vi "collisionTest.vi"(0 "Game in":refnum<class "Game.lvclass">, 1 "TestParameters":T7, 2 "replace active":bool, 3 "Dest_array":T8(array[cluster]), 4 "grSIM replacement":T4, 5 "error in (no error)":errorcluster) -> (14 "Game out":refnum<class "Game.lvclass">, 15 "TestTeam":refnum<class "Ally.lvclass">, 16 "replaceRobots":bool, 17 "grSIM replacement out":T4, 18 "State":T1 {"progress" scale=0.0..100.0}, 19 "error out":errorcluster)   [LabVIEW 2020, in "Game.lvclass"]
uses:
  Game.lvclass
  Controls/grSimReplacement.ctl
  Communication_class/Paths/grSim Packet Command UDP Test Folder/grSim/grSim RobotReplacement.ctl
  Communication_class/Paths/grSim Packet Command UDP Test Folder/grSim/grSim_BallReplacement.ctl
  Ally_class/Ally.lvclass
  C:/Users/anton/Desktop/RoboIME/SSL_AI/Team_class/Team.lvclass
  VelocityPlanningTest/Controls/velocityPlanningState.ctl
  VelocityPlanningTest/Controls/trajectoryState.ctl
  Controls/RobotModelTestState.ctl
  Game.lvclass/Game.ctl
  Team_class/Team.lvclass/Team.ctl
  Object_class/Object.lvclass/Object.ctl
  Robot_class/Robot.lvclass/Robot.ctl
  <vilib>/Analysis/1siggen.llb/Ramp Pattern by Samples.vi
  <vilib>/Analysis/_algsub.llb/Real Vector Norm.vi
  Read AllyRef.vi
  Team_class/Read RobotRef.vi
  Object_class/Read x.vi
  Object_class/Read y.vi
  Read EnemyRef.vi
  Robot_class/Write dest_x.vi
  Robot_class/Write dest_y.vi
  Team_class/Write RobotRef.vi
  Robot_class/Robot.lvclass
  C:/Users/anton/Desktop/RoboIME/SSL_AI/Object_class/Object.lvclass
  Enemy_class/Enemy.lvclass
  Utilities_class/Utilities.lvclass
  <vilib>/Analysis/NI_AALPro.lvlib
  <vilib>/Analysis/NI_AALBase.lvlib
panel:
  out "velocityPlanningState":T2={"est_vel"=0.0, "dist_to_(Dest/L)"=0.0, "V0_model"=0.0, "max_dist_to_break"=0.0, "v_sent"=0.0, "traj_state"=enum."replace"}
  out "XY Graph":cluster{"Ramp Pattern":dbl[], i32[]}(graph)
  out "Array 2":dbl[](array[numeric])
  out "Array":i32[](array[numeric])
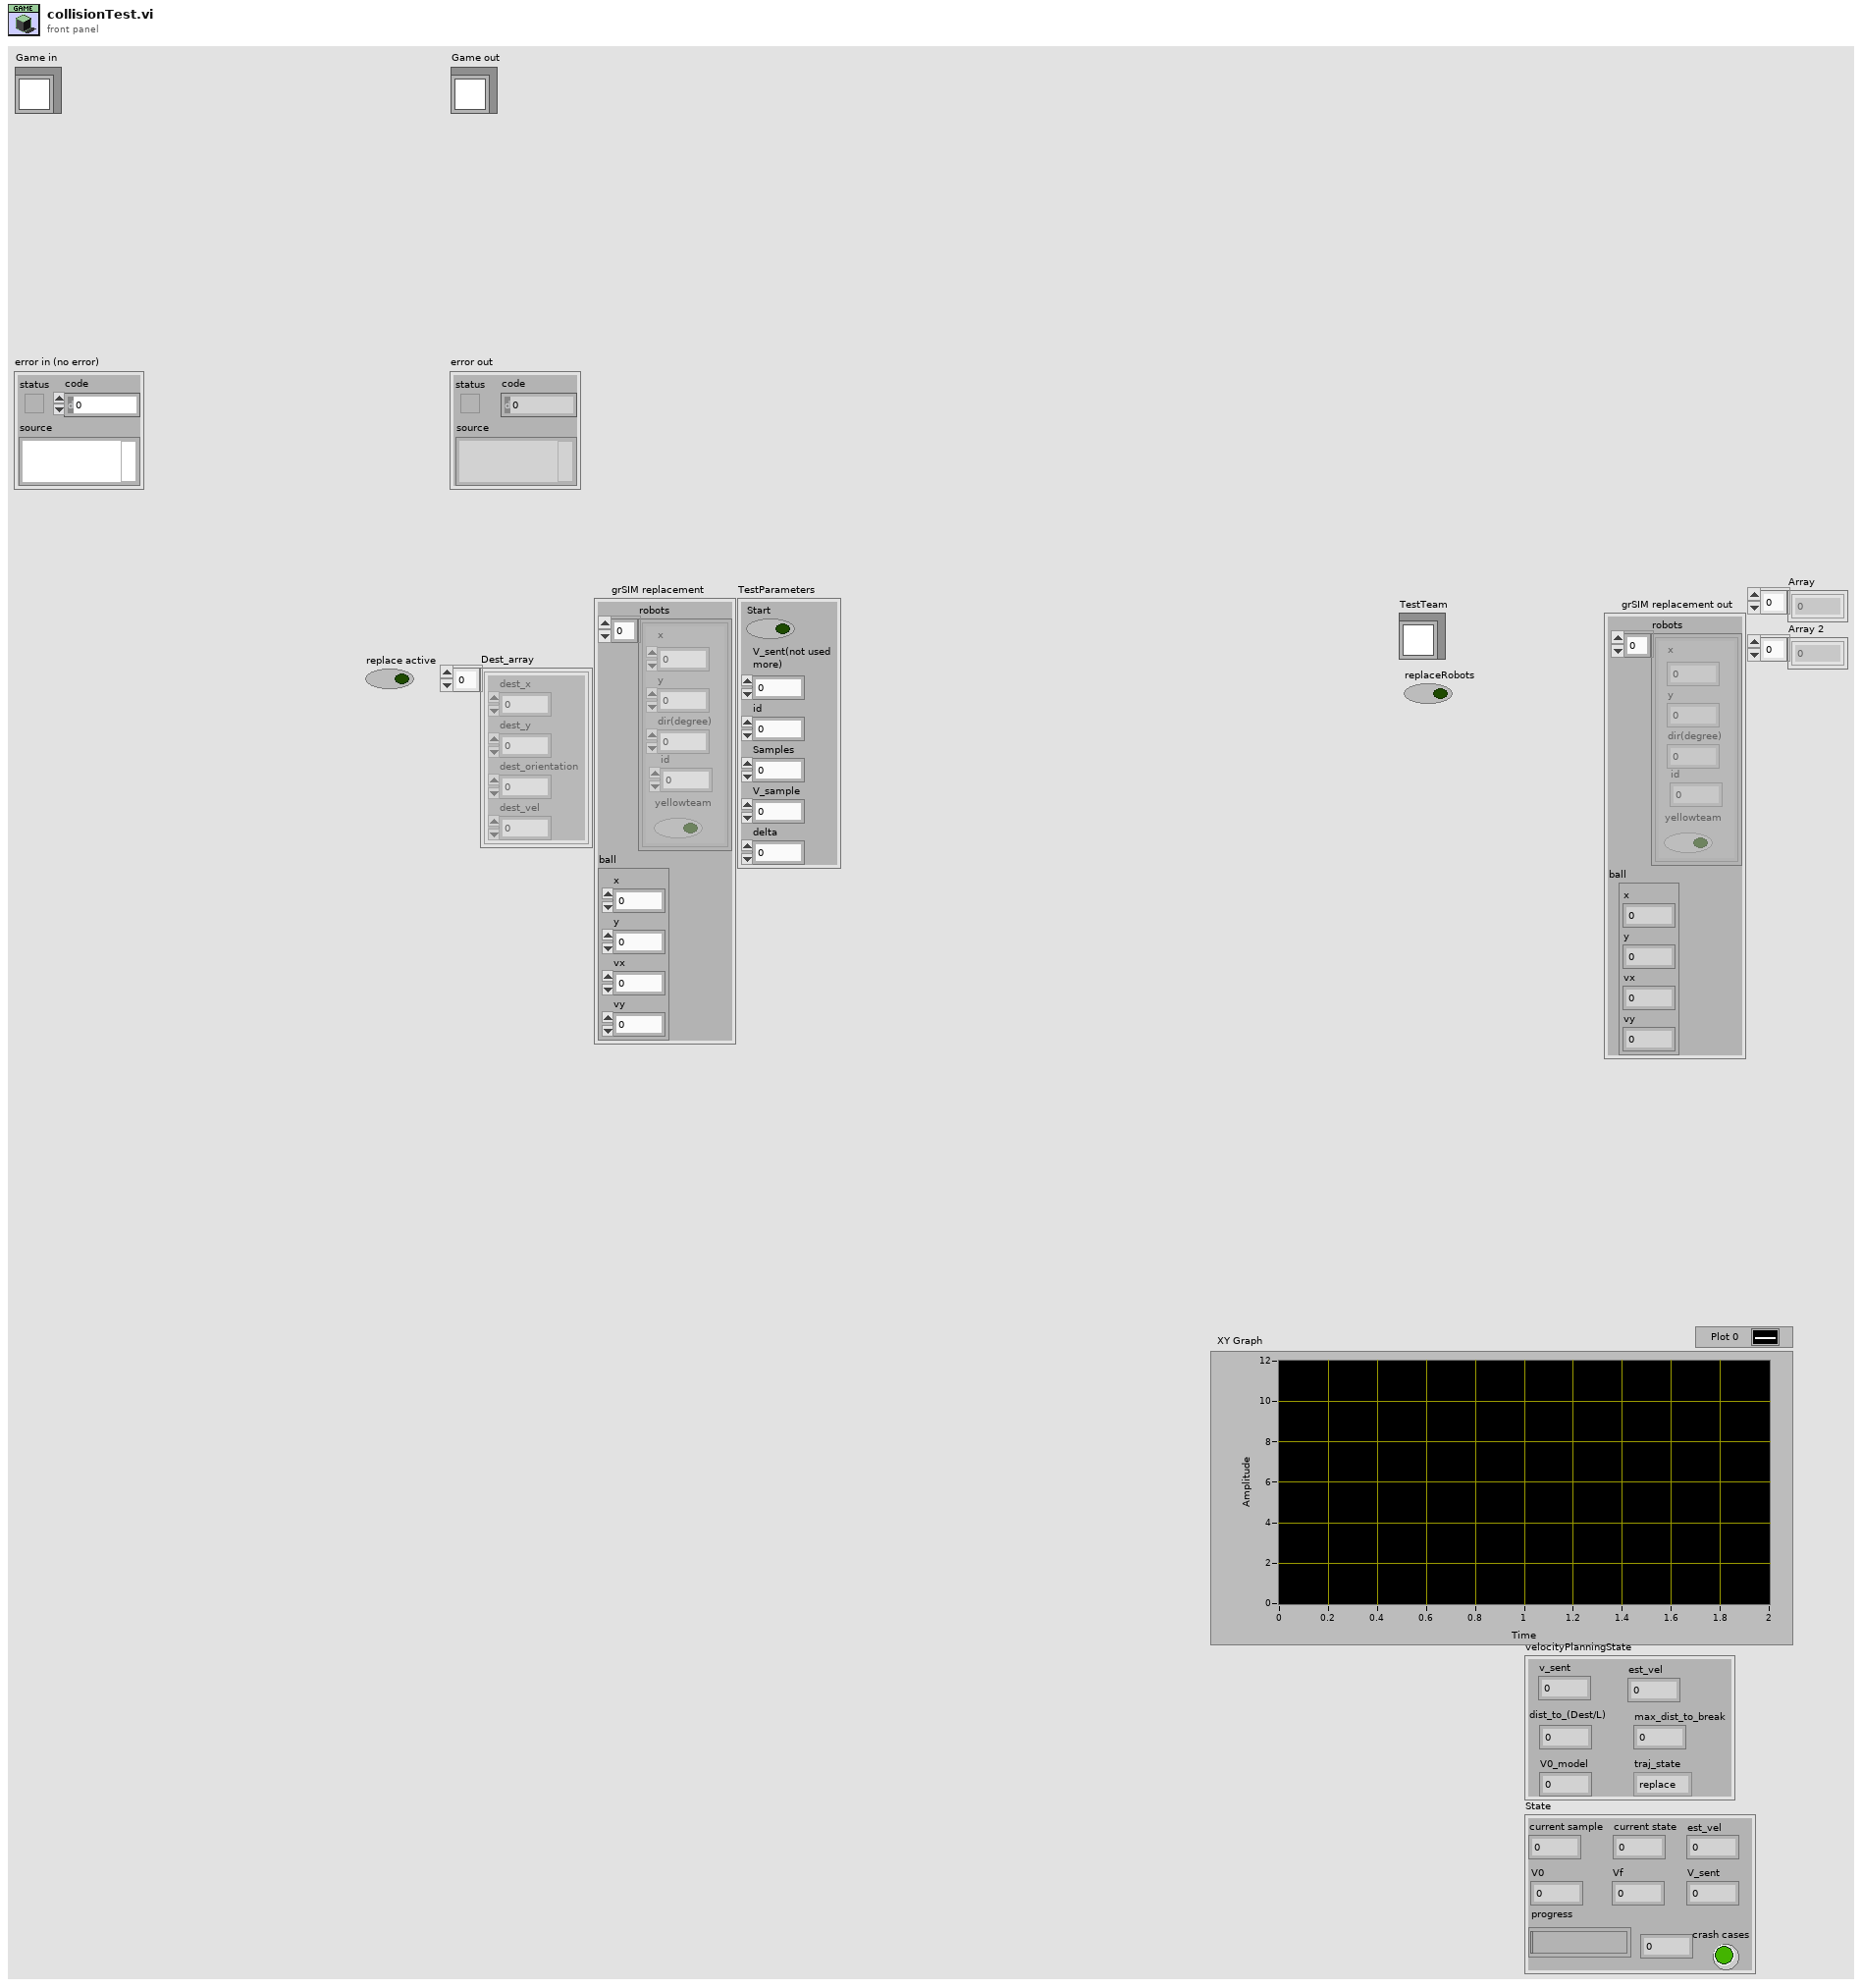
[diagram p1: front panel]
types:
  T1 = typedef "RobotModelTestState.ctl" = cluster{"current sample":i32, "V0":dbl, "Vf":dbl, "progress":dbl, "current state":i32, "est_vel":dbl, "V_sent":dbl, "crash cases":bool}
  T2 = typedef "velocityPlanningState.ctl" = cluster{"est_vel":dbl, "dist_to_(Dest/L)":dbl, "V0_model":dbl, "max_dist_to_break":dbl, "v_sent":dbl, "traj_state":T3}
  T3 = typedef "trajectoryState.ctl" = enum16{"stop", "replace", "circle", "line"}
  T4 = typedef "grSimReplacement.ctl" = cluster{"robots":T5[], "ball":T6}
  T5 = typedef "grSim RobotReplacement.ctl" = cluster{"x":dbl, "y":dbl, "dir(degree)":dbl, "yellowteam":bool, "id":u32}
  T6 = typedef "grSim_BallReplacement.ctl" = cluster{"x":dbl, "y":dbl, "vx":dbl, "vy":dbl}
  T7 = cluster{"Start":bool, "V_sent(not used\nmore)":dbl, "id":i32, "Samples":dbl, "V_sample":dbl, "delta":dbl}
  T8 = cluster{"dest_x":dbl, "dest_y":dbl, "dest_orientation":dbl, "dest_vel":dbl}[]
  T9 = enum16{"Finish", "Replace", "Collide", "Move", "Crash"}
  T10 = cluster{"dest_x":dbl, "dest_y":dbl, "dest_orientation":dbl, "dest_vel":dbl}
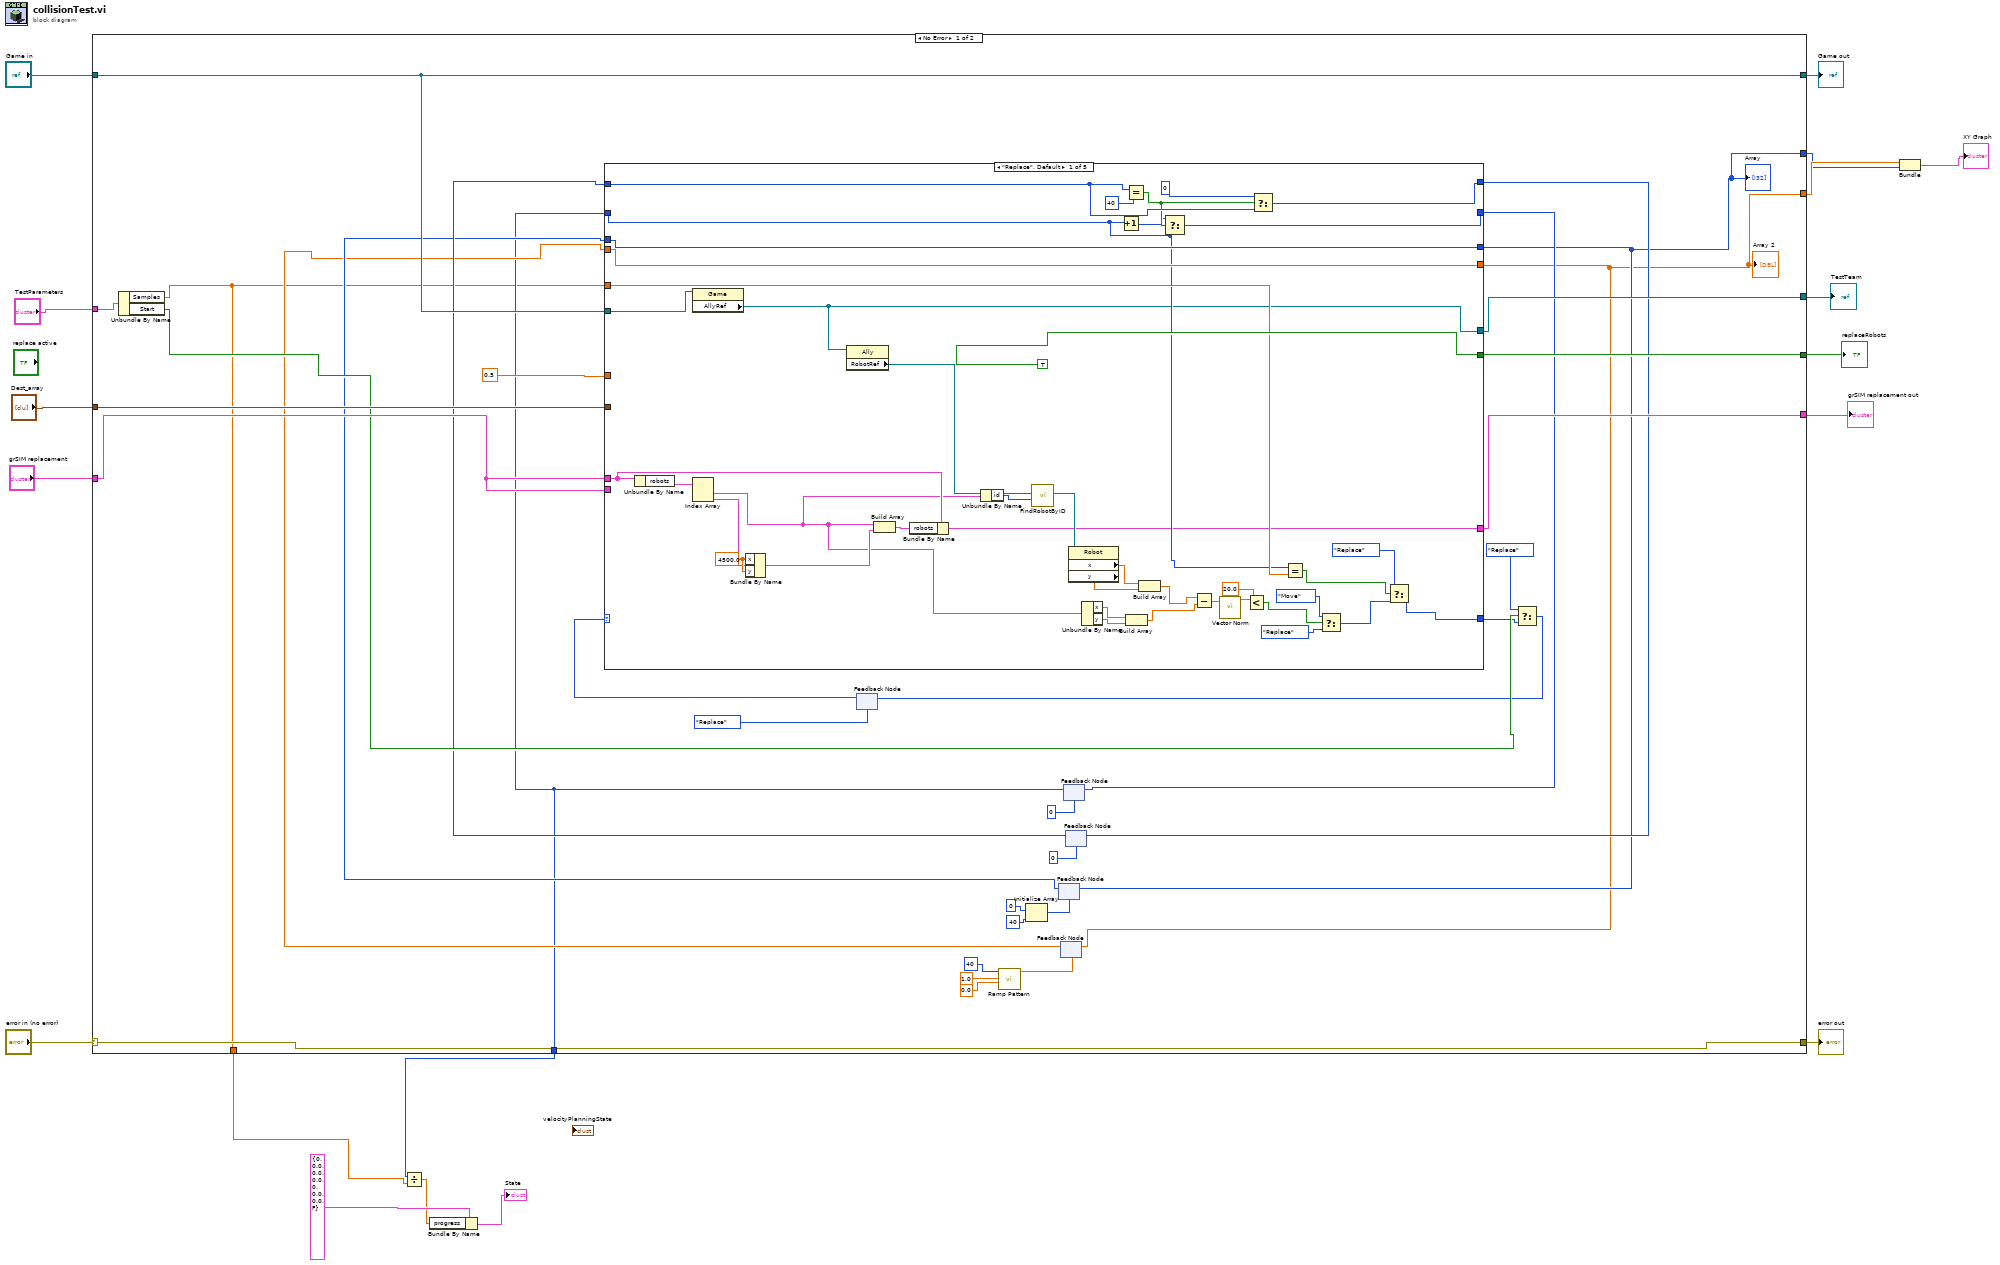
[diagram p0: block diagram]
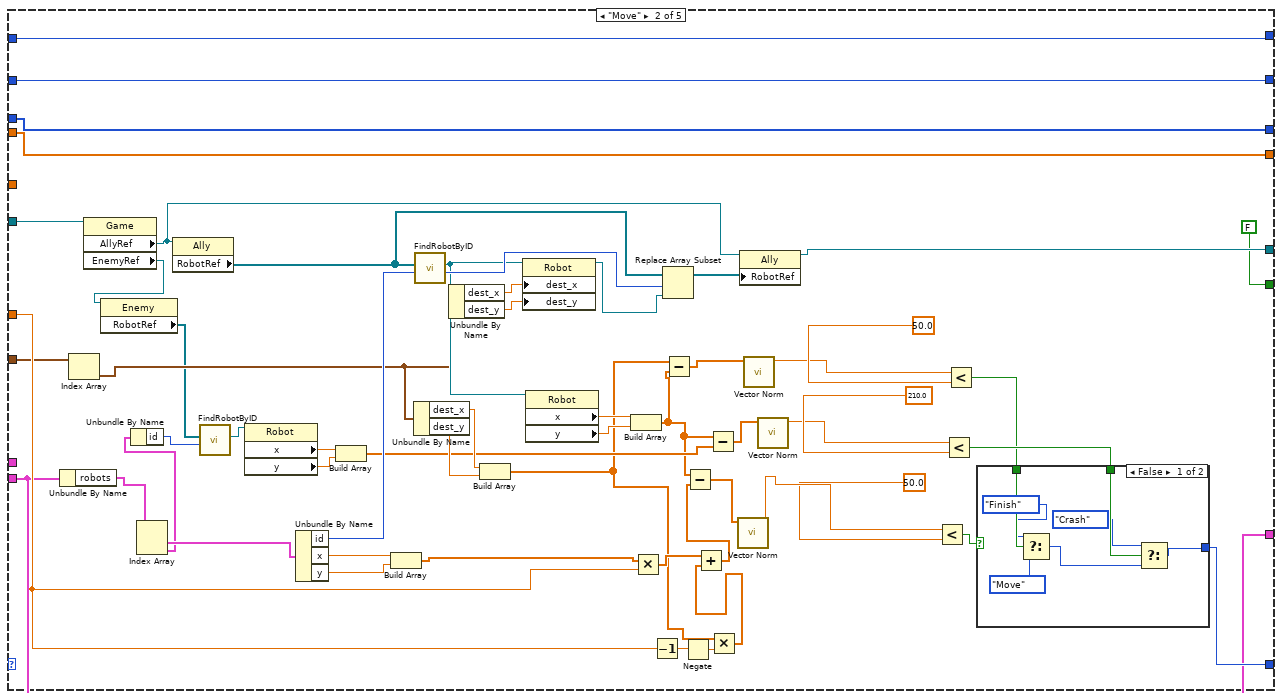
[diagram p2: hidden frame]
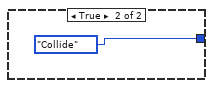
[diagram p3: hidden frame]
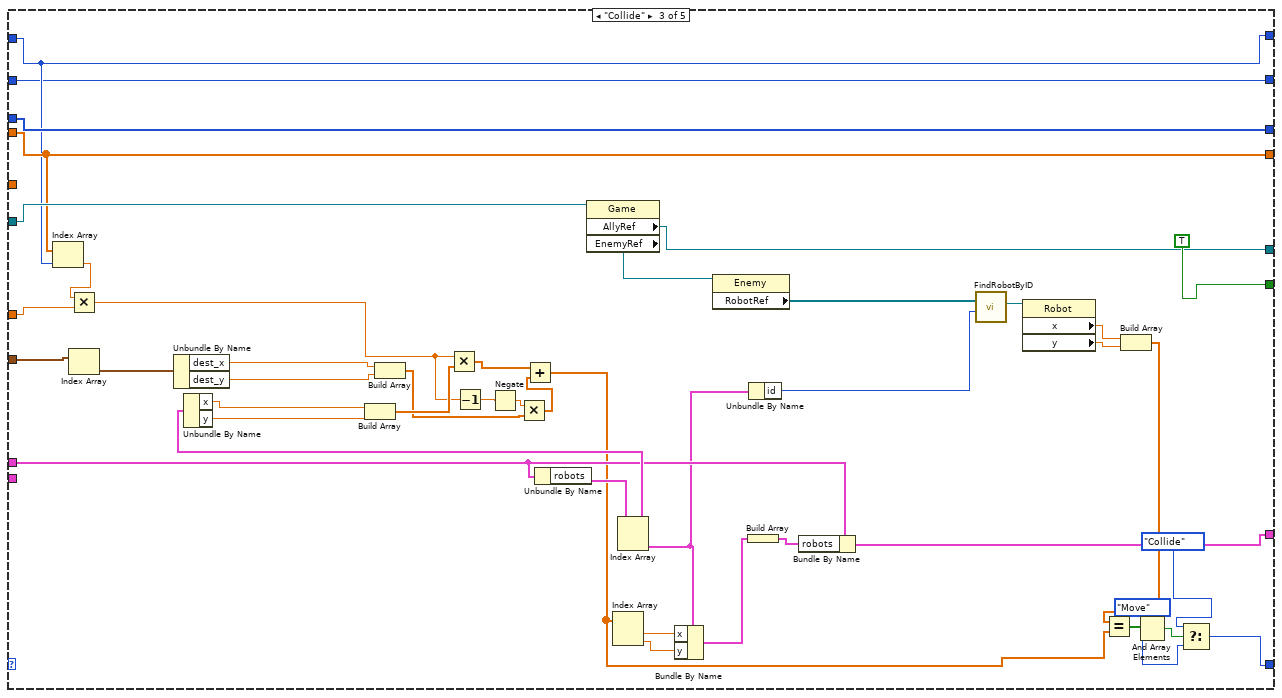
[diagram p4: hidden frame]
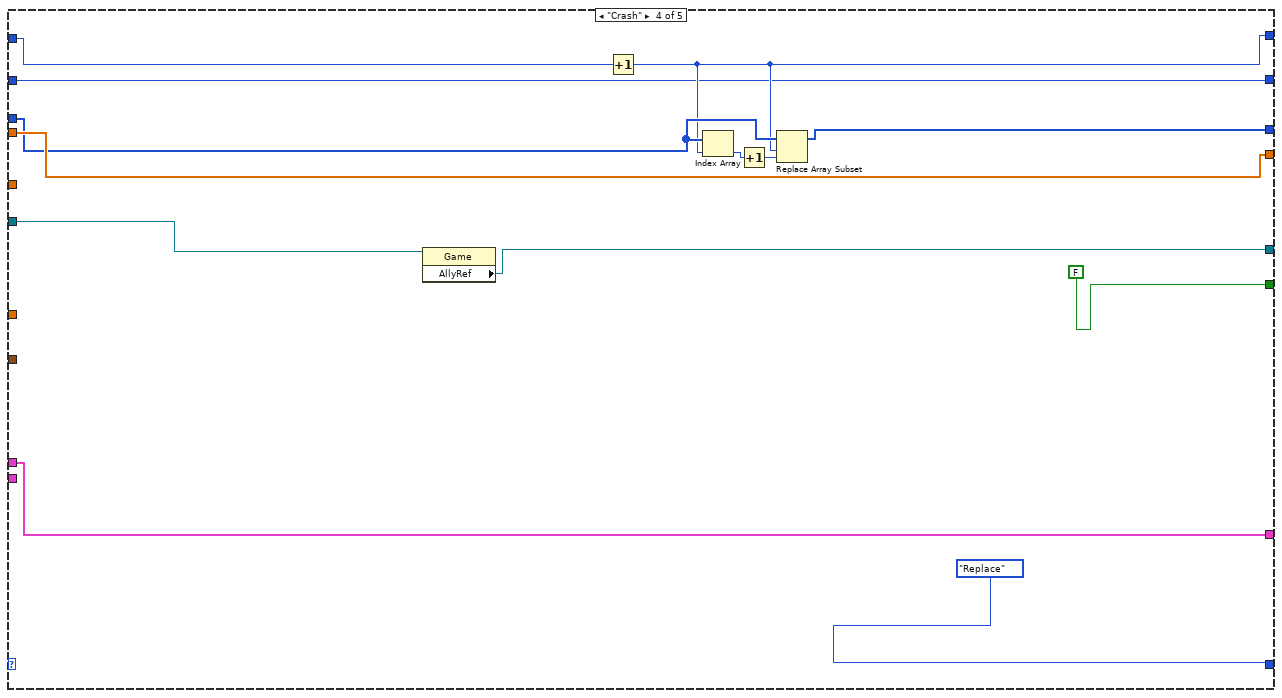
[diagram p5: hidden frame]
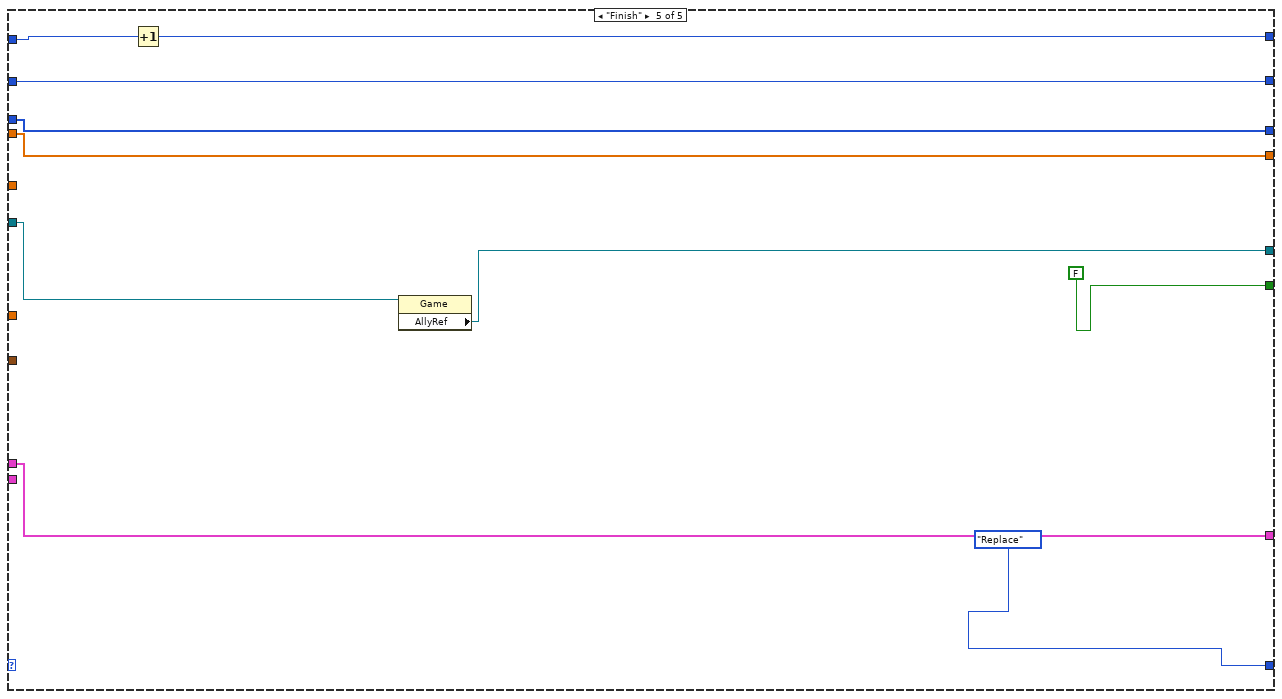
[diagram p6: hidden frame]
diagram:
  n1 = case shown="No Error" "error in (no error)" {
    selector: "error in (no error)" -> [w51 w226]
    tunnel: [w51 w226] -> w17
    tunnel: [w48 w225] -> w15
    tunnel: "Game in" -> [w48 w225]
    tunnel: [w50 _] -> w14
    tunnel: "grSIM replacement" -> [w45 _]
    tunnel: [w49 _] -> w12
    tunnel: "Dest_array" -> [w47 _]
    tunnel: [w46 _] -> w10
    tunnel: "TestParameters" -> [w44 _]
    tunnel: [w22 _] -> w6
    tunnel: [w21 _] -> w7
    tunnel: [w20 _] -> w4
    tunnel: [w19 _] -> w3
    frame No Error {
      n2 = Unbundle By Name(w44) -> ("Samples"=w19:dbl, "Start"=w43:bool)
      n3 = feedback #1(T9."Replace") -> (w36:T9)
      n4 = call-poly <vilib>:"Ramp Pattern.vi"("start"=0.0, "end"=1.0, "samples"=40) -> ("Ramp Pattern"=w27:dbl[])  [unwired: 7 in, 1 out]
      n5 = Initialize Array(0 ("dimension size"), 40 ("dimension size")) -> (w28:i32[])
      n6 = feedback #2(w28) -> (w26:i32[])
      n7 = feedback #3(w27) -> (w25:dbl[])
      n8 = feedback #4(0) -> (w20:i32)
      n9 = feedback #5(0) -> (w29:i32)
      n10 = case shown="\"Replace\", Default" w36 {
        tunnel: [w80 w131 w163 T9."Replace" T9."Replace"] -> w34
        tunnel: [TRUE FALSE TRUE FALSE FALSE] -> w50
        tunnel: w45 -> [w86 _ w182 w210 w220]
        tunnel: [w66 w112 w198 w210 w220] -> w49
        tunnel: w48 -> [w87 w149 w184 w213 w223]
        tunnel: w47 -> [_ w117 w178 _ _]
        tunnel: [w69 w144 w183 w212 w222] -> w46
        tunnel: w45 -> [_ w112 _ _ _]
        tunnel: [w84 w96 w162 w204 w217] -> w22
        tunnel: [w83 w95 w161 w208 w216] -> w21
        tunnel: 0.5 -> [_ w126 w181 _ _]
        tunnel: w29 -> [w78 w97 w160 w209 w219]
        tunnel: [w76 w97 w160 w203 w218] -> w31
        tunnel: w26 -> [w84 w96 w162 w207 w217]
        tunnel: w25 -> [w83 w95 w161 w208 w216]
        tunnel: w20 -> [w71 w94 w158 w202 w215]
        tunnel: [w75 w94 w158 w202 w215] -> w23
        tunnel: w19 -> [w73 _ _ _ _]
        frame "Replace", Default {
          w89 = 4500.0
          n11 = Unbundle By Name(w86) -> ("robots"=w91:T5[])
          n12 = property class="Game"(reference=w87) -> ("AllyRef"=w69:refnum<class "Ally.lvclass">)  [unwired: 1 in, 2 out]
          n13 = Index Array(array=w91) -> (element #1=w65:T5, element #2=w85:T5)  [unwired: 2 in]
          n14 = Bundle By Name(cluster=w85, "x"=w89, "y"=w89) -> (w88:T5)
          n15 = property class="Ally"(reference=w69) -> ("RobotRef"=w68:refnum<class "Robot.lvclass">[])  [unwired: 1 in, 2 out]
          n16 = Build Array(w65, w88) -> (w90:T5[])
          n17 = Bundle By Name(cluster=w86, "robots"=w90) -> (w66:T4)
          n18 = Unbundle By Name(w65) -> ("id"=w70:u32)
          n19 = call "FindRobotByID.vi"("id"=w70, "RobotRef"=w68) -> ("Robot"=w67:refnum<class "Robot.lvclass">)  [unwired: 6 in, 3 out]
          n20 = property class="Robot"(reference=w67) -> ("x"=w62:dbl, "y"=w61:dbl)  [unwired: 1 in, 2 out]
          n21 = Unbundle By Name(w65) -> ("x"=w64:dbl, "y"=w63:dbl)
          n22 = Increment(x=w71) -> (x+1=w74:i32)
          n23 = Equal?(x=w78, y=40) -> (x = y?=w77:bool)
          n24 = Build Array(w64, w63) -> (w56:dbl[])
          n25 = Build Array(w62, w61) -> (w57:dbl[])
          n26 = Select(t=w74, s=w77, f=w71) -> (s? t:f=w75:i32)
          n27 = Subtract(x=w57, y=w56) -> (x-y=w55:dbl[])
          n28 = call-poly <vilib>:"Vector Norm.vi"("Input Vector"=w55) -> ("norm"=w54:dbl)  [unwired: 9 in, 1 out]
          n29 = Less?(x=w54, y=20.0) -> (x < y?=w52:bool)
          n30 = Select(t=0 ("y"), s=w77, f=w78) -> (s? t:f=w76:i32)
          n31 = Equal?(x=w71, y=w73) -> (x = y?=w72:bool)
          n32 = Select(t=T9."Move", s=w52, f=T9."Replace") -> (s? t:f=w58:T9)
          n33 = Select(t=T9."Replace", s=w72, f=w58) -> (s? t:f=w80:T9)
        }
        frame "Move" {
          n34 = Unbundle By Name(w112) -> ("robots"=w142:T5[])
          n35 = Index Array(array=w117) -> (element=w115:T10)  [unwired: 1 in]
          n36 = property class="Game"(reference=w149) -> ("AllyRef"=w146:refnum<class "Ally.lvclass">, "EnemyRef"=w111:refnum<class "Enemy.lvclass">)  [unwired: 1 in, 2 out]
          n37 = property class="Enemy"(reference=w111) -> ("RobotRef"=w110:refnum<class "Robot.lvclass">[])  [unwired: 1 in, 2 out]
          n38 = Index Array(array=w142) -> (element #1=w143:T5, element #2=w109:T5)  [unwired: 2 in]
          n39 = Unbundle By Name(w109) -> ("id"=w108:u32)
          n40 = property class="Ally"(reference=w146) -> ("RobotRef"=w139:refnum<class "Robot.lvclass">[])  [unwired: 1 in, 2 out]
          n41 = call "FindRobotByID.vi"("id"=w108, "RobotRef"=w110) -> ("Robot"=w107:refnum<class "Robot.lvclass">)  [unwired: 6 in, 3 out]
          n42 = property class="Robot"(reference=w107) -> ("x"=w106:dbl, "y"=w105:dbl)  [unwired: 1 in, 2 out]
          n43 = Unbundle By Name(w143) -> ("id"=w141:u32, "x"=w120:dbl, "y"=w119:dbl)
          n44 = Build Array(w106, w105) -> (w104:dbl[])
          n45 = Build Array(w120, w119) -> (w118:dbl[])
          n46 = Unbundle By Name(w115) -> ("dest_x"=w114:dbl, "dest_y"=w113:dbl)
          n47 = call "FindRobotByID.vi"("id"=w141, "RobotRef"=w139) -> ("index"=w148:i32, "Robot"=w138:refnum<class "Robot.lvclass">)  [unwired: 6 in, 2 out]
          n48 = Unbundle By Name(w115) -> ("dest_x"=w116:dbl, "dest_y"=w93:dbl)
          n49 = Build Array(w114, w113) -> (w102:dbl[])
          n50 = property class="Robot"(reference=w138, "dest_x"=w116, "dest_y"=w93) -> (reference out=w147:refnum<class "Robot.lvclass">)  [unwired: 1 in, 1 out]
          n51 = property class="Robot"(reference=w138) -> ("x"=w137:dbl, "y"=w136:dbl)  [unwired: 1 in, 2 out]
          n52 = Build Array(w137, w136) -> (w103:dbl[])
          n53 = Multiply(x=w118, y=w126) -> (x*y=w123:dbl[])
          n54 = Decrement(x=w126) -> (x-1=w125:dbl)
          n55 = Replace Array Subset(array=w139, new element=w147, index=w148) -> (w145:refnum<class "Robot.lvclass">[])
          n56 = Subtract(x=w102, y=w103) -> (x-y=w101:dbl[])
          n57 = Negate(x=w125) -> (-x=w124:dbl)
          n58 = Subtract(x=w103, y=w104) -> (x-y=w130:dbl[])
          n59 = Multiply(x=w102, y=w124) -> (x*y=w122:dbl[])
          n60 = Add(x=w123, y=w122) -> (x+y=w121:dbl[])
          n61 = Subtract(x=w103, y=w121) -> (x-y=w135:dbl[])
          n62 = call-poly <vilib>:"Vector Norm.vi"("Input Vector"=w135) -> ("norm"=w134:dbl)  [unwired: 9 in, 1 out]
          n63 = property class="Ally"(reference=w146, "RobotRef"=w145) -> (reference out=w144:refnum<class "Ally.lvclass">)  [unwired: 1 in, 1 out]
          n64 = call-poly <vilib>:"Vector Norm.vi"("Input Vector"=w101) -> ("norm"=w99:dbl)  [unwired: 9 in, 1 out]
          n65 = call-poly <vilib>:"Vector Norm.vi"("Input Vector"=w130) -> ("norm"=w128:dbl)  [unwired: 9 in, 1 out]
          n66 = Less?(x=w134, y=50.0) -> (x < y?=w132:bool)
          n67 = Less?(x=w128, y=210.0) -> (x < y?=w127:bool)
          n68 = Less?(x=w99, y=50.0) -> (x < y?=w98:bool)
          n69 = case shown="False" w132 {
            tunnel: [w154 T9."Collide"] -> w131
            tunnel: w127 -> [w156 _]
            tunnel: w98 -> [w153 _]
            frame False {
              n70 = Select(t=T9."Finish", s=w153, f=T9."Move") -> (s? t:f=w150:T9)
              n71 = Select(t=T9."Crash", s=w156, f=w150) -> (s? t:f=w154:T9)
            }
            frame True {
            }
          }
        }
        frame "Collide" {
          n72 = Index Array(array=w161, index=w160) -> (element=w159:dbl)
          n73 = Multiply(x=w159, y=w181) -> (x*y=w180:dbl)
          n74 = Index Array(array=w178) -> (element=w177:T10)  [unwired: 1 in]
          n75 = Unbundle By Name(w177) -> ("dest_x"=w195:dbl, "dest_y"=w194:dbl)
          n76 = Build Array(w195, w194) -> (w179:dbl[])
          n77 = Decrement(x=w180) -> (x-1=w188:dbl)
          n78 = Negate(x=w188) -> (-x=w187:dbl)
          n79 = Multiply(x=w187, y=w179) -> (x*y=w189:dbl[])
          n80 = Unbundle By Name(w182) -> ("robots"=w201:T5[])
          n81 = property class="Game"(reference=w184) -> ("AllyRef"=w183:refnum<class "Ally.lvclass">, "EnemyRef"=w176:refnum<class "Enemy.lvclass">)  [unwired: 1 in, 2 out]
          n82 = Index Array(array=w201) -> (element #1=w196:T5, element #2=w175:T5)  [unwired: 2 in]
          n83 = Unbundle By Name(w196) -> ("x"=w192:dbl, "y"=w193:dbl)
          n84 = Build Array(w192, w193) -> (w191:dbl[])
          n85 = Multiply(x=w180, y=w191) -> (x*y=w190:dbl[])
          n86 = Add(x=w190, y=w189) -> (x+y=w168:dbl[])
          n87 = Index Array(array=w168) -> (element #1=w186:dbl, element #2=w185:dbl)  [unwired: 2 in]
          n88 = Bundle By Name(cluster=w175, "x"=w186, "y"=w185) -> (w197:T5)
          n89 = property class="Enemy"(reference=w176) -> ("RobotRef"=w174:refnum<class "Robot.lvclass">[])  [unwired: 1 in, 2 out]
          n90 = Build Array(w197) -> (w200:T5[])
          n91 = Unbundle By Name(w175) -> ("id"=w173:u32)
          n92 = Bundle By Name(cluster=w182, "robots"=w200) -> (w198:T4)
          n93 = call "FindRobotByID.vi"("id"=w173, "RobotRef"=w174) -> ("Robot"=w172:refnum<class "Robot.lvclass">)  [unwired: 6 in, 3 out]
          n94 = property class="Robot"(reference=w172) -> ("x"=w171:dbl, "y"=w170:dbl)  [unwired: 1 in, 2 out]
          n95 = Build Array(w171, w170) -> (w169:dbl[])
          n96 = Equal?(x=w169, y=w168) -> (x = y?=w167:bool[])
          n97 = And Array Elements(Boolean array=w167) -> (logical AND=w166:bool)
          n98 = Select(t=T9."Collide", s=w166, f=T9."Move") -> (s? t:f=w163:T9)
        }
        frame "Crash" {
          n99 = property class="Game"(reference=w213) -> ("AllyRef"=w212:refnum<class "Ally.lvclass">)  [unwired: 1 in, 2 out]
          n100 = Increment(x=w209) -> (x+1=w203:i32)
          n101 = Index Array(array=w207, index=w203) -> (element=w206:i32)
          n102 = Increment(x=w206) -> (x+1=w205:i32)
          n103 = Replace Array Subset(array=w207, new element=w205, index=w203) -> (w204:i32[])
        }
        frame "Finish" {
          n104 = Increment(x=w219) -> (x+1=w218:i32)
          n105 = property class="Game"(reference=w223) -> ("AllyRef"=w222:refnum<class "Ally.lvclass">)  [unwired: 1 in, 2 out]
        }
      }
      "Array" <- w22
      "Array 2" <- w21
      n106 = feedback-in #2(w22) -> ()
      n107 = feedback-in #3(w21) -> ()
      n108 = feedback-in #4(w23) -> ()
      n109 = feedback-in #5(w31) -> ()
      n110 = Select(t=T9."Replace", s=w43, f=w34) -> (s? t:f=w32:T9)
      n111 = feedback-in #1(w32) -> ()
    }
    frame Error {
    }
  }
  "error out" <- w17
  "Game out" <- w15
  "TestTeam" <- w10
  "grSIM replacement out" <- w12
  "replaceRobots" <- w14
  n112 = Divide(x=w4, y=w3) -> (x/y=w2:dbl)
  n113 = Bundle By Name(cluster=T1 {"current sample"=0, "V0"=0.0, "Vf"=0.0, "progress"=0.0, "current state"=0, "est_vel"=0.0, "V_sent"=0.0, "crash cases"=FALSE} ("State"), "progress"=w2) -> (→"State":T1)
  n114 = Bundle("Ramp Pattern"=w7, w6) -> (→"XY Graph":cluster{"Ramp Pattern":dbl[], i32[]})  [unwired: 1 in]
